vi "Start.vi"(8 "error in (no error)":errorcluster, 9 "FadeRate":dbl, 10 "FadePicture":u32[][](array[numeric]), 11 "FadeOutTiles in":refnum<class "FadeOutTiles.lvclass">) -> (0 "error out":errorcluster, 3 "FadeOutTiles out":refnum<class "FadeOutTiles.lvclass">)   [LabVIEW 2019, in "RT_Game.lvlib" / "FadeOutTiles.lvclass"]
uses:
  FadeOutTiles.lvclass
  FadeOutTiles.lvclass/FadeOutTiles.ctl
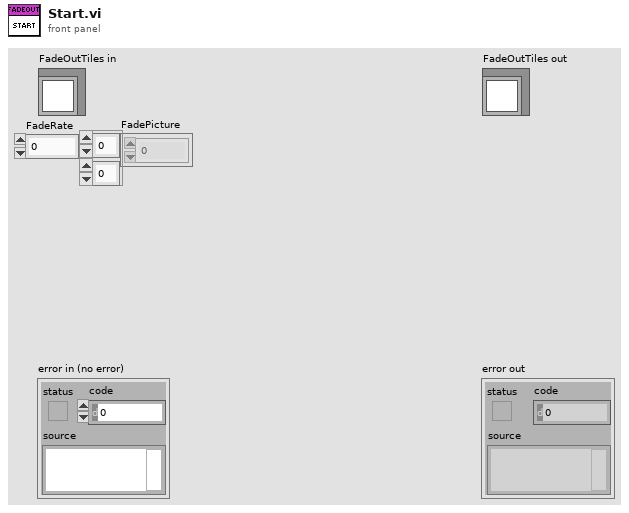
[diagram p1: front panel]
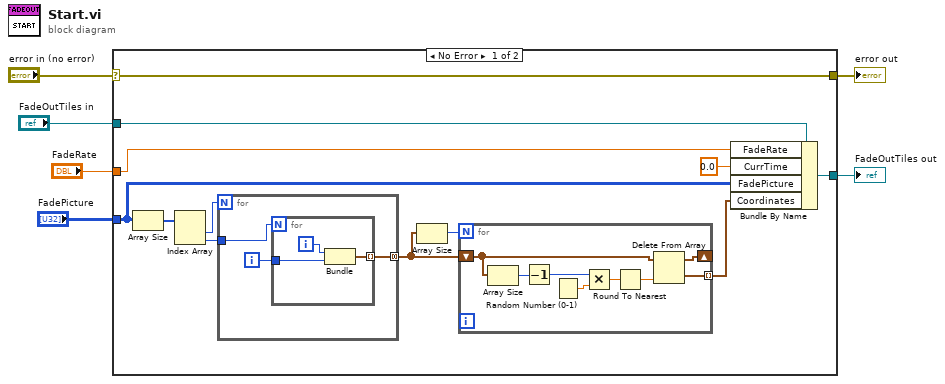
[diagram p0: block diagram]
diagram:
  n1 = case shown="No Error" "error in (no error)" {
    selector: "error in (no error)" -> [w17 w34]
    tunnel: [w17 w34] -> w5
    tunnel: [w16 w33] -> w3
    tunnel: "FadeOutTiles in" -> [w18 w33]
    tunnel: "FadePicture" -> [w13 _]
    tunnel: "FadeRate" -> [w14 _]
    frame No Error {
      n2 = Array Size(array=w13) -> (size(s)=w12:i32[])
      n3 = Index Array(array=w12) -> (element #1=w11:i32, element #2=w10:i32)  [unwired: 2 in]
      n4 = for {
        N: w11 -> [_]
        tunnel: w10 -> [w29]
        tunnel: [w27] -> w8 mode=concatenating
        i -> [w28]
        n5 = for {
          N: w29 -> [_]
          tunnel: w28 -> [w31]
          tunnel: [w30] -> w27 mode=indexing
          i -> [w32]
          n6 = Bundle(w32, w31) -> (w30:cluster{i32, i32})  [unwired: 1 in]
        }
      }
      n7 = Array Size(array=w8) -> (size(s)=w7:i32)
      n8 = for {
        N: w7 -> [_]
        shift-right: [w26] -> _
        shift-left: w8 -> [w25]
        tunnel: [w19] -> w9 mode=indexing
        n9 = Array Size(array=w25) -> (size(s)=w24:i32)
        n10 = Decrement(x=w24) -> (x-1=w23:i32)
        n11 = Random Number (0-1)() -> (number: 0 to 1=w22:dbl)
        n12 = Multiply(x=w23, y=w22) -> (x*y=w21:dbl)
        n13 = Round To Nearest(number=w21) -> (nearest integer value=w20:dbl)
        n14 = Delete From Array(array=w25, index=w20) -> (deleted portion=w19:cluster{i32, i32}, array with subset deleted=w26:cluster{i32, i32}[])  [unwired: 1 in]
      }
      n15 = Bundle By Name(cluster=w18, "FadeRate"=w14, "CurrTime"=0.0, "FadePicture"=w13, "Coordinates"=w9) -> (w16:refnum<class "FadeOutTiles.lvclass">)
    }
    frame Error {
    }
  }
  "error out" <- w5
  "FadeOutTiles out" <- w3
